vi "Write startIsTrue.vi"(10 "startIsTrue":bool, 11 "ApplicationHandler in":refnum<class "ApplicationHandler.lvclass">) -> (3 "ApplicationHandler out":refnum<class "ApplicationHandler.lvclass">)   [LabVIEW 2013, in "ComponentData.lvlib" / "ApplicationHandler.lvclass"]
uses:
  <userlib>/Common/Component/Application/RT/ComponentData/ApplicationHandler/ApplicationHandler.lvclass
  <userlib>/Common/Component/Application/RT/ComponentData/ApplicationHandler/ApplicationHandler.lvclass/ApplicationHandler.ctl
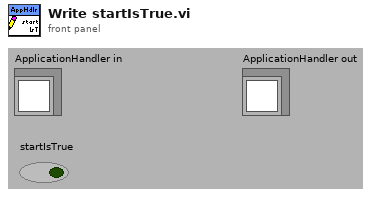
[diagram p1: front panel]
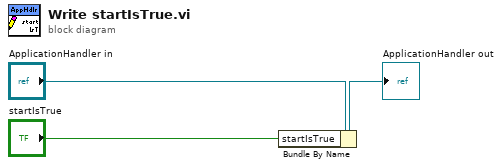
[diagram p0: block diagram]
diagram:
  n1 = Bundle By Name(cluster="ApplicationHandler in", "startIsTrue"="startIsTrue") -> (→"ApplicationHandler out":refnum<class "ApplicationHandler.lvclass">)
